vi "Configure Modulation (Wideband IQ).vi"(0 "VISA resource name":refnum<visa-resource-name>, 1 "Enable Wideband I/Q Modulation (T:Enable)":bool=TRUE, 5 "Enable Wideband I/Q Adjustment (F:Disable)":bool, 7 "I Channel Offset Value (0 percent)":dbl, 9 "Q Channel Offset Value (0 percent)":dbl, 11 "error in (no error)":errorcluster, 12 "Quadrature Skew (0 deg)":dbl) -> (4 "VISA resource name out":refnum<visa-resource-name>, 15 "error out":errorcluster)   [LabVIEW 2014, in "Agilent PSG MXG Series.lvlib"]
doc: "Configures the wideband I/Q modulator and the wideband I/Q adjustments.\n\n<B>Notes:</B>\n(1) This VI is valid only in E8267C, E8267D.\n\n(2) For E8267C, this VI is valid only when the instrument installs <B>Option 002</B> (Internal baseband generator) or <B>Option 602</B> (Digital bus baseband generator), and <B>Option 015</B> (Wideband external I/Q inputs).\n\n(3) For E8267D, this VI is valid only when the instrument installs <B>Option 601</B> or <B>Option 602</B> (Internal baseband generator), and <B>Option 015</B>."
uses:
  Agilent PSG MXG Series.lvlib
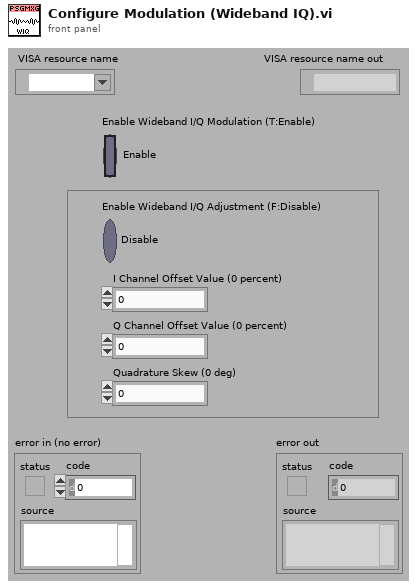
[diagram p1: front panel]
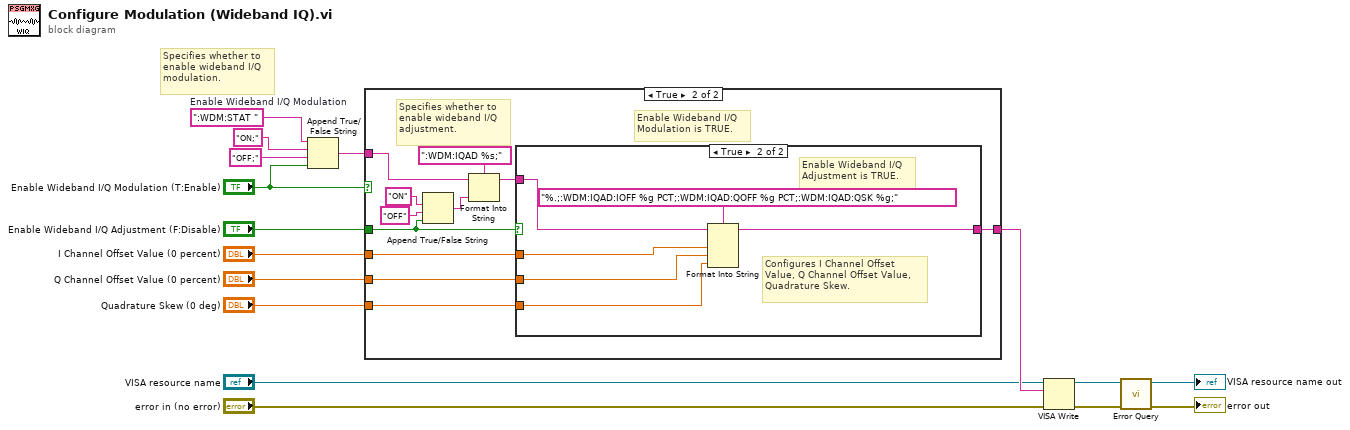
[diagram p0: block diagram]
diagram:
  w16 = ":WDM:STAT "  # Enable Wideband I/Q Modulation
  # "Specifies whether to\nenable wideband I/Q\nmodulation."
  n1 = Append True/False String(1:"Enable Wideband I/Q Modulation (T:Enable)", 2:"OFF;" ("false string"), 3:"ON;" ("true string"), 4:w16) -> (0:w13:string)
  n2 = case shown="True" "Enable Wideband I/Q Modulation (T:Enable)" {
    tunnel: w13 -> [w17 w28]
    tunnel: "Enable Wideband I/Q Adjustment (F:Disable)" -> [_ w24]
    tunnel: "I Channel Offset Value (0 percent)" -> [_ w22]
    tunnel: "Q Channel Offset Value (0 percent)" -> [_ w21]
    tunnel: "Quadrature Skew (0 deg)" -> [_ w20]
    tunnel: [w17 w19] -> w7
    frame False {
      # "Enable Wideband I/Q\nModulation is FALSE."
    }
    frame True {
      # "Specifies whether to\nenable wideband I/Q\nadjustment."
      # "Enable Wideband I/Q\nModulation is TRUE."
      n3 = Append True/False String(1:w24, 2:"OFF" ("false string"), 3:"ON" ("true string")) -> (0:w26:string)  [unwired: 1 out]
      n4 = Format Into String(format string=":WDM:IQAD %s;", initial string=w28, w26) -> (resulting string=w23:string)  [unwired: 1 in, 1 out]
      n5 = case shown="True" w24 {
        tunnel: w23 -> [w29 w34]
        tunnel: w22 -> [_ w33]
        tunnel: w21 -> [_ w32]
        tunnel: w20 -> [_ w31]
        tunnel: [w29 w30] -> w19
        frame False {
          # "Enable Wideband I/Q\nAdjustment is FALSE."
        }
        frame True {
          # "Configures I Channel Offset\nValue, Q Channel Offset Value,\nQuadrature Skew."
          # "Enable Wideband I/Q\nAdjustment is TRUE."
          n6 = Format Into String(format string="%.;:WDM:IQAD:IOFF %g PCT;:WDM:IQAD:QOFF %g PCT;:WDM:IQAD:QSK %g;", initial string=w34, w33, w32, w31) -> (resulting string=w30:string)  [unwired: 1 in, 1 out]
        }
      }
    }
  }
  n7 = VISA Write(VISA resource name="VISA resource name", write buffer=w7, error in (no error)="error in (no error)") -> (VISA resource name out=w6:refnum<visa-resource-name>, error out=w5:errorcluster)  [unwired: 1 out]
  n8 = call "Error Query.vi"("error in (no error)"=w5, "VISA resource name"=w6) -> ("error out"=→"error out":errorcluster, "VISA resource name out"=→"VISA resource name out":refnum<visa-resource-name>)  [unwired: 8 out]
